vi "Set Power.vi"(8 "error in (no error)":errorcluster, 9 "Power":dbl, 11 "Coherent Laser in":refnum<class "Coherent Laser.lvclass">) -> (0 "error out":errorcluster, 3 "Coherent Laser out":refnum<class "Coherent Laser.lvclass">)   [LabVIEW 2023, in "Coherent Laser.lvlib" / "Coherent Laser.lvclass"]
uses:
  Coherent Laser.lvclass
  Coherent Laser.lvclass/Coherent Laser.ctl
  Coherent Laser.lvlib
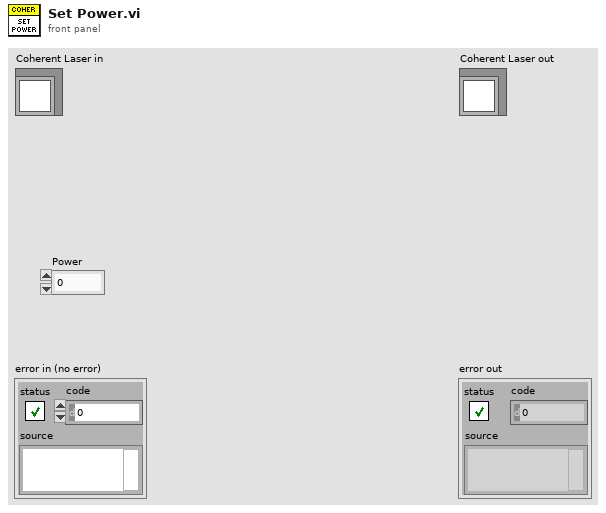
[diagram p1: front panel]
types:
  T1 = enum16{"Disable", "Laser Quantum", "Coherent OBIS", "PRM1-Z8", "Coherent HOPS"}
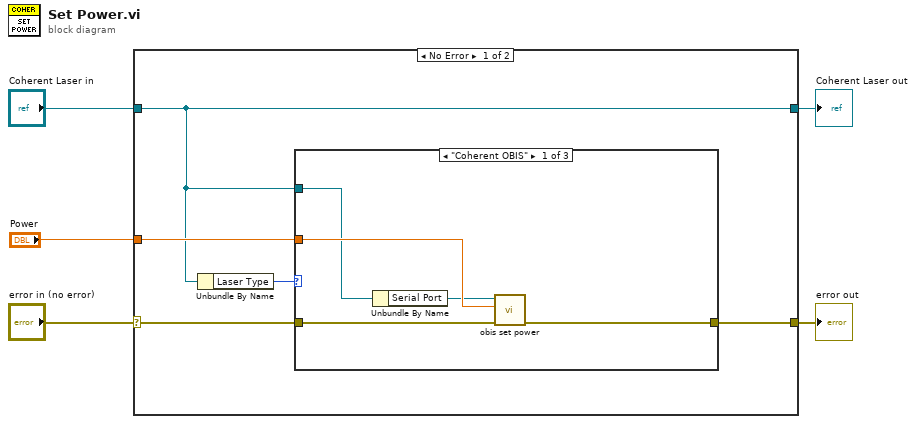
[diagram p0: block diagram]
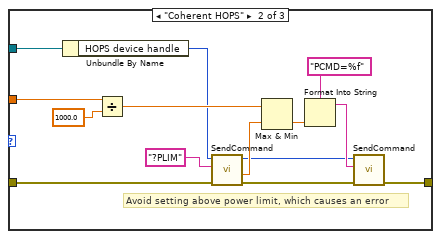
[diagram p2: hidden frame]
diagram:
  n1 = case shown="No Error" "error in (no error)" {
    selector: "error in (no error)" -> [w9 w32]
    tunnel: [w8 w32] -> w4
    tunnel: [w6 w31] -> w2
    tunnel: "Coherent Laser in" -> [w6 w31]
    tunnel: "Power" -> [w7 _]
    frame No Error {
      n2 = Unbundle By Name(w6) -> ("Laser Type"=w10:T1)
      n3 = case shown="\"Coherent OBIS\"" w10 {
        tunnel: w9 -> [w15 w22 w30]
        tunnel: w7 -> [w13 w28 _]
        tunnel: [w14 w24 w30] -> w8
        tunnel: w6 -> [w11 w29 _]
        frame "Coherent OBIS" {
          n4 = Unbundle By Name(w11) -> ("Serial Port"=w12:refnum<visa-resource-name>)
          n5 = call "obis set power.vi"("error in"=w15, "Power"=w13, "Serial Port"=w12) -> ("error out"=w14:errorcluster)  [unwired: 7 in, 1 out]
        }
        frame "Coherent HOPS" {
          # "Avoid setting above power limit, which causes an error"
          n6 = Unbundle By Name(w29) -> ("HOPS device handle"=w17:u64)
          n7 = Divide(x=w28, y=1000.0) -> (x/y=w20:dbl)
          n8 = call "SendCommand.vi"("error in"=w22, "Command"="?PLIM", "Device Handle"=w17) -> ("error out"=w21:errorcluster, "Number"=w19:dbl, "Dup Handle"=w16:u64)  [unwired: 3 in, 1 out]
          n9 = Max & Min(x=w20, y=w19) -> (min(x,y)=w18:dbl)  [unwired: 1 out]
          n10 = Format Into String(format string="PCMD=%f" ("Command"), w18) -> (resulting string=w25:string)  [unwired: 2 in, 1 out]
          n11 = call "SendCommand.vi"("error in"=w21, "Command"=w25, "Device Handle"=w16) -> ("error out"=w24:errorcluster)  [unwired: 3 in, 3 out]
        }
        frame Default {
        }
      }
    }
    frame Error {
    }
  }
  "error out" <- w4
  "Coherent Laser out" <- w2
